vi "AI IRQ Initialize.vi"() -> (14 "Fatal Error Out":T11, 15 "State Out":T1)   [LabVIEW 2021, in "myRIO Register AI IRQ.xnode"]
uses:
  <vilib>/myRIO/Instrument Drivers/IRQ/IO IRQ/vis/myRIO Register AI IRQ.xnode
  <vilib>/XNodeSupport/XNodeErrorCluster.ctl
  <vilib>/myRIO/Instrument Drivers/IRQ/IO IRQ/vis/AI IRQ State.ctl
  <vilib>/myRIO/Common/Instrument Driver Framework/Utilities/typedefs/myRIOXPeripheral.ctl
  <vilib>/XNodeSupport/XNodeTerm4Array.ctl
  <vilib>/XNodeSupport/XNodeTerm4.ctl
  <vilib>/XNodeSupport/XNodeString.ctl
  <vilib>/XNodeSupport/XNodeVariant.ctl
  <vilib>/XNodeSupport/XNodeRect32.ctl
  <vilib>/XNodeSupport/XNodeInt.ctl
  <vilib>/XNodeSupport/XNodeBool.ctl
  <vilib>/XNodeSupport/XNodeTermDirection.ctl
  <vilib>/myRIO/Common/Instrument Driver Framework/myRIO v1.0/IRQ/typedefs/AI IRQ Type.ctl
  <vilib>/myRIO/Common/Instrument Driver Framework/myRIO v1.0/IRQ/typedefs/Callback VI Ref.ctl
  <vilib>/myRIO/Common/Instrument Driver Framework/Utilities/vis/myRIOXGlobal.vi
  <vilib>/XNodeSupport/NI_XNodeSupport.lvlib
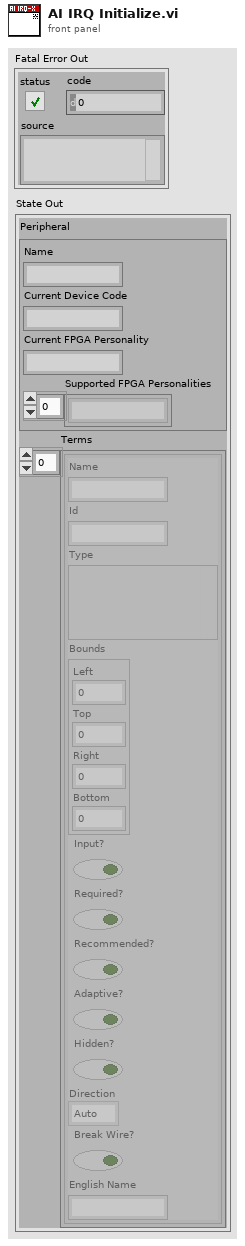
[diagram p1: front panel]
types:
  T1 = typedef "myRIO Register AI IRQ.xnode/AI IRQ State.ctl" = cluster{"Peripheral":T2, "Terms":T3}
  T2 = typedef "myRIOXPeripheral.ctl" = cluster{"Name":string, "Current Device Code":string, "Current FPGA Personality":string, "Supported FPGA Personalities":string[]}
  T3 = typedef "NI_XNodeSupport.lvlib/XNodeTerm4Array.ctl" = T4[]
  T4 = typedef "NI_XNodeSupport.lvlib/XNodeTerm4.ctl" = cluster{"Name":T5, "Id":T5, "Type":T6, "Bounds":T7, "Input?":T9, "Required?":T9, "Recommended?":T9, "Adaptive?":T9, "Hidden?":T9, "Direction":T10, "Break Wire?":T9, "English Name":T5}
  T5 = typedef "NI_XNodeSupport.lvlib/XNodeString.ctl" = string
  T6 = typedef "NI_XNodeSupport.lvlib/XNodeVariant.ctl" = variant
  T7 = typedef "NI_XNodeSupport.lvlib/XNodeRect32.ctl" = cluster{"Left":T8, "Top":T8, "Right":T8, "Bottom":T8}
  T8 = typedef "NI_XNodeSupport.lvlib/XNodeInt.ctl" = i32
  T9 = typedef "NI_XNodeSupport.lvlib/XNodeBool.ctl" = bool
  T10 = typedef "NI_XNodeSupport.lvlib/XNodeTermDirection.ctl" = enum32{"Auto", "Up", "Down", "Left", "Right", "Center"}
  T11 = typedef "NI_XNodeSupport.lvlib/XNodeErrorCluster.ctl" = errorcluster
  T12 = typedef "AI IRQ Type.ctl" = enum16{"Analog falling edge", "Analog rising edge"}
  T13 = typedef "Callback VI Ref.ctl" = refnum<vi>
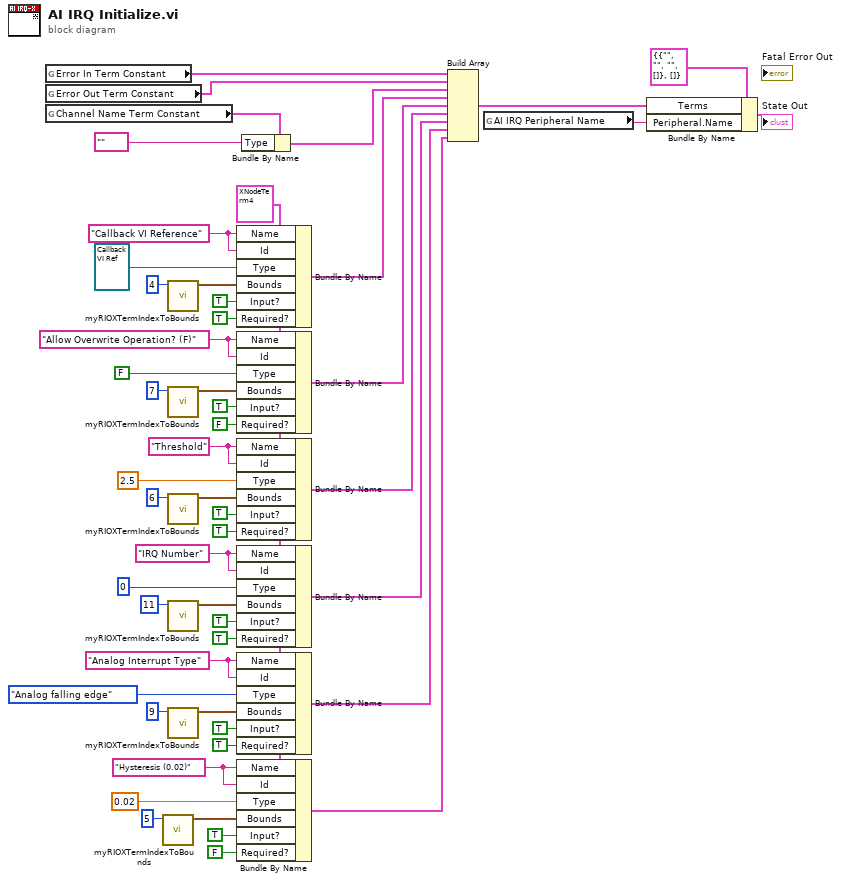
[diagram p0: block diagram]
diagram:
  w6 = T5 "Hysteresis (0.02)" ("Name")
  w21 = T5 "Analog Interrupt Type" ("Name")
  w23 = T5 "IRQ Number" ("Name")
  w29 = T5 "Threshold" ("Name")
  w37 = T5 "Allow Overwrite Operation? (F)" ("Name")
  w44 = T5 "Callback VI Reference" ("Name")
  w2 = T4 {"Name"="", "Id"="", "Type"=variant, "Bounds"={"Left"=0, "Top"=0, "Right"=0, "Bottom"=0}, "Input?"=FALSE, "Required?"=FALSE, "Recommended?"=FALSE, "Adaptive?"=FALSE, "Hidden?"=FALSE, "Direction"=enum."Auto", "Break Wire?"=FALSE, "English Name"=""} ("Error In Term Constant")
  n1 = global read "myRIOXGlobal.vi" "Error In Term Constant"() -> (w49:T4)
  n2 = global read "myRIOXGlobal.vi" "Error Out Term Constant"() -> (w48:T4)
  n3 = global read "myRIOXGlobal.vi" "Channel Name Term Constant"() -> (w13:T4)
  n4 = call <vilib>:"myRIOXTermIndexToBounds.vi"("Index"=5) -> ("Bounds"=w4:T7)  [unwired: 10 in]
  n5 = call <vilib>:"myRIOXTermIndexToBounds.vi"("Index"=4) -> ("Bounds"=w47:T7)  [unwired: 10 in]
  n6 = call <vilib>:"myRIOXTermIndexToBounds.vi"("Index"=7) -> ("Bounds"=w34:T7)  [unwired: 10 in]
  n7 = call <vilib>:"myRIOXTermIndexToBounds.vi"("Index"=6) -> ("Bounds"=w27:T7)  [unwired: 10 in]
  n8 = call <vilib>:"myRIOXTermIndexToBounds.vi"("Index"=11) -> ("Bounds"=w24:T7)  [unwired: 10 in]
  n9 = call <vilib>:"myRIOXTermIndexToBounds.vi"("Index"=9) -> ("Bounds"=w20:T7)  [unwired: 10 in]
  n10 = Bundle By Name(cluster=w2, "Name"=w44, "Id"=w44, "Type"=T13 refnum ("Callback VI"), "Bounds"=w47, "Input?"=T9 TRUE, "Required?"=T9 TRUE) -> (w42:T4)
  n11 = Bundle By Name(cluster=w2, "Name"=w37, "Id"=w37, "Type"=FALSE ("Allow Overwrite? (F)"), "Bounds"=w34, "Input?"=T9 TRUE, "Required?"=T9 FALSE) -> (w41:T4)
  n12 = Bundle By Name(cluster=w2, "Name"=w29, "Id"=w29, "Type"=2.5 ("Threshold"), "Bounds"=w27, "Input?"=T9 TRUE, "Required?"=T9 TRUE) -> (w40:T4)
  n13 = Bundle By Name(cluster=w2, "Name"=w23, "Id"=w23, "Type"=u8 0 ("IRQ Number"), "Bounds"=w24, "Input?"=T9 TRUE, "Required?"=T9 TRUE) -> (w39:T4)
  n14 = Bundle By Name(cluster=w2, "Name"=w21, "Id"=w21, "Type"=AI_IRQ_Type."Analog falling edge" ("AI IRQ Type"), "Bounds"=w20, "Input?"=T9 TRUE, "Required?"=T9 TRUE) -> (w38:T4)
  n15 = Bundle By Name(cluster=w2, "Name"=w6, "Id"=w6, "Type"=0.02 ("Threshold"), "Bounds"=w4, "Input?"=T9 TRUE, "Required?"=T9 FALSE) -> (w1:T4)
  n16 = Bundle By Name(cluster=w13, "Type"=tag "" ("myRIO AI IRQ Channel")) -> (w12:T4)
  n17 = Build Array(w49, w48, w12, w42, w41, w40, w39, w38, w1) -> (w11:T4[])
  n18 = global read "myRIOXGlobal.vi" "AI IRQ Peripheral Name"() -> (w50:string)
  n19 = Bundle By Name(cluster=T1 {"Peripheral"={"Name"="", "Current Device Code"="", "Current FPGA Personality"="", "Supported FPGA Personalities"=[]}, "Terms"=[]} ("State Out"), "Terms"=w11, "Peripheral.Name"=w50) -> (→"State Out":T1)
